vi "New.vi"(8 "error in (no error)":errorcluster, 11 "ChannelMap":map{string, refnum<data-value>}(c390)) -> (0 "error out":errorcluster, 2 "callback UEs":T1, 3 "plot handle":refnum<class "NIringPlotHandle.lvclass">)   [LabVIEW 2021, in "NIringPlotHandle.lvclass"]
uses:
  NIringPlotHandle.lvclass
  <vilib>/National Instruments/Variant Ring Buffer/Ring Buffer.lvclass
  NIringPlotHandle.lvclass/NIringPlotHandle.ctl
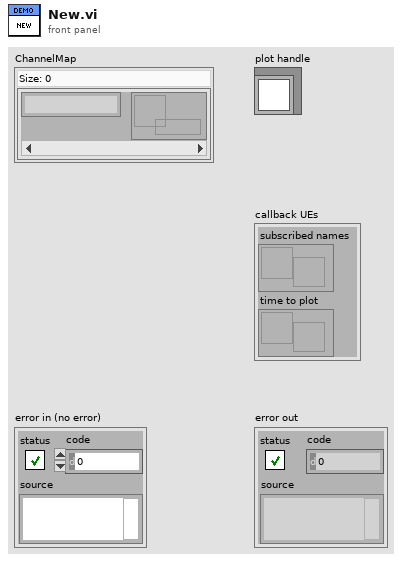
[diagram p1: front panel]
types:
  T1 = cluster{"subscribed names":refnum<user-event>, "time to plot":refnum<user-event>}
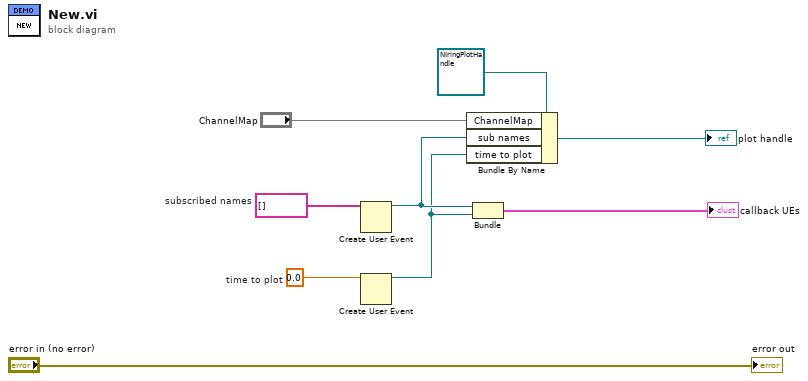
[diagram p0: block diagram]
diagram:
  w7 = 0.0  # time to plot
  w8 = string[] []  # subscribed names
  n1 = Create User Event(user event datatype=w8) -> (user event=w6:refnum<user-event>)  [unwired: 1 in, 1 out]
  n2 = Create User Event(user event datatype=w7) -> (user event=w5:refnum<user-event>)  [unwired: 1 in, 1 out]
  n3 = Bundle By Name(cluster=refnum<class "NIringPlotHandle.lvclass"> refnum ("BluePlotDemo.lvlib:BluePlotHandleDemo.lvclass"), "ChannelMap"="ChannelMap", "sub names"=w6, "time to plot"=w5) -> (→"plot handle":refnum<class "NIringPlotHandle.lvclass">)
  n4 = Bundle("subscribed names"=w6, "time to plot"=w5) -> (→"callback UEs":T1)  [unwired: 1 in]
  "error out" <- "error in (no error)"
